vi "Launch UI.vi"(8 "error in (no error)":errorcluster, 11 "UI Controller in":refnum<class "Controller.lvclass">) -> (0 "error out":errorcluster, 3 "UI Controller out":refnum<class "Controller.lvclass">)   [LabVIEW 2016, in "Controller Actor.lvlib" / "Controller.lvclass"]
uses:
  <userlib>/Common Components/Controller/Controller.lvclass
  C:/Program Files (x86)/National Instruments/LabVIEW 2016/vi.lib/ActorFramework/Actor/Actor.lvclass
  <userlib>/Common Components/Controller UI/Controller UI.lvclass
  C:/Program Files (x86)/National Instruments/LabVIEW 2016/user.lib/Common Components/User Interface/UI.lvclass
  <userlib>/Common Components/Controller/Controller.lvclass/Controller.ctl
  <userlib>/Common Components/User Interface/UI.lvclass/UI.ctl
  <vilib>/ActorFramework/Actor/Actor.lvclass/Actor.ctl
  <vilib>/ActorFramework/Message Enqueuer/Message Enqueuer.lvclass/Message Enqueuer.ctl
  <userlib>/Common Components/User Interface/Accessors/Write Hide me.vi
  <vilib>/ActorFramework/Message Enqueuer/Init from Existing Queue.vi
  <vilib>/ActorFramework/Message Enqueuer/Message Enqueuer.lvclass
  <vilib>/ActorFramework/Actor/Actor.lvclass
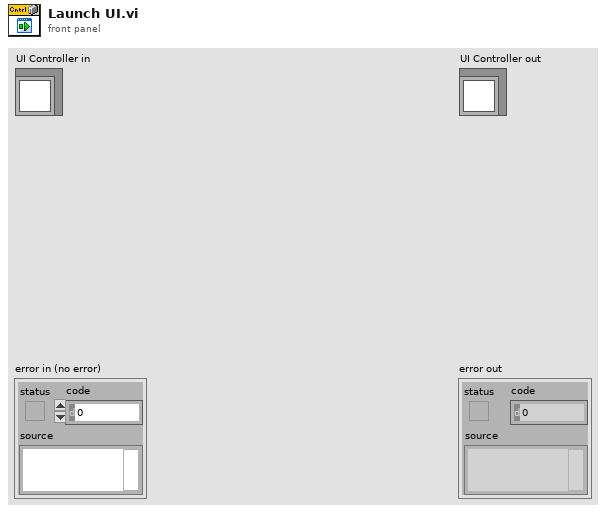
[diagram p1: front panel]
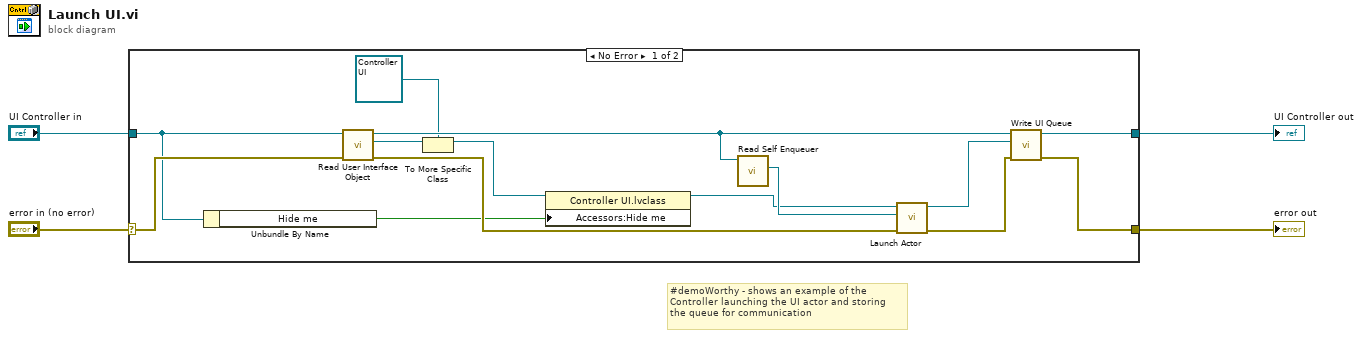
[diagram p0: block diagram]
diagram:
  # "#demoWorthy - shows an example of the \nController launching the UI actor and storing\nthe queue for communication"
  n1 = case shown="No Error" "error in (no error)" {
    selector: "error in (no error)" -> [w12 w20]
    tunnel: [w10 w20] -> w3
    tunnel: [w17 w19] -> w1
    tunnel: "UI Controller in" -> [w8 w19]
    frame No Error {
      n2 = Unbundle By Name(w8) -> ("Hide me"=w7:bool)
      n3 = call <userlib>:"Read User Interface Object.vi"("error in (no error)"=w12, "UI Controller in"=w8) -> ("error out"=w13:errorcluster, "UI.lvclass"=w15:refnum<class "UI.lvclass">, "UI Controller out"=w14:refnum<class "Controller.lvclass">)  [unwired: 7 in]
      n4 = To More Specific Class(target class=refnum<class "Controller UI.lvclass"> refnum ("Controller UI.lvlib:Controller UI.lvclass"), reference=w15) -> (specific class reference=w6:refnum<class "Controller UI.lvclass">)  [unwired: 1 in, 1 out]
      n5 = property class="Controller UI.lvclass"(reference=w6, "Accessors:Hide me"=w7) -> (reference out=w9:refnum<class "Controller UI.lvclass">)  [unwired: 1 in, 1 out]
      n6 = call <vilib>:"Read Self Enqueuer.vi"("Actor"=w14) -> ("Self Enqueuer"=w16:refnum<class "Message Enqueuer.lvclass">)  [unwired: 10 in]
      n7 = call <vilib>:"Launch Actor.vi"("error in (no error)"=w13, "Actor-to-Caller Enqueuer"=w16, "Actor"=w9) -> ("error out"=w11:errorcluster, "Caller-To-Actor Enqueuer"=w18:refnum<class "Message Enqueuer.lvclass">)  [unwired: 7 in]
      n8 = call <userlib>:"Write UI Queue.vi"("error in (no error)"=w11, "UI Queue"=w18, "UI Controller in"=w14) -> ("error out"=w10:errorcluster, "UI Controller out"=w17:refnum<class "Controller.lvclass">)  [unwired: 7 in]
    }
    frame Error {
    }
  }
  "error out" <- w3
  "UI Controller out" <- w1
